vi "Log.vi"(10 "Log Packet":T1, 11 "LVQueue Sink in":refnum<class "LVQueue Sink.lvclass">) -> (0 "error out":errorcluster, 3 "LVQueue Sink out":refnum<class "LVQueue Sink.lvclass">)   [LabVIEW 2019, in "LVQueue Sink.lvclass"]
uses:
  LVQueue Sink.lvclass
  Composed Log/Types/Log Packet.ctl
  Composed Log/Types/Log Level.ctl
  LVQueue Sink.lvclass/LVQueue Sink.ctl
  Composed Log/Composed Log.lvlib
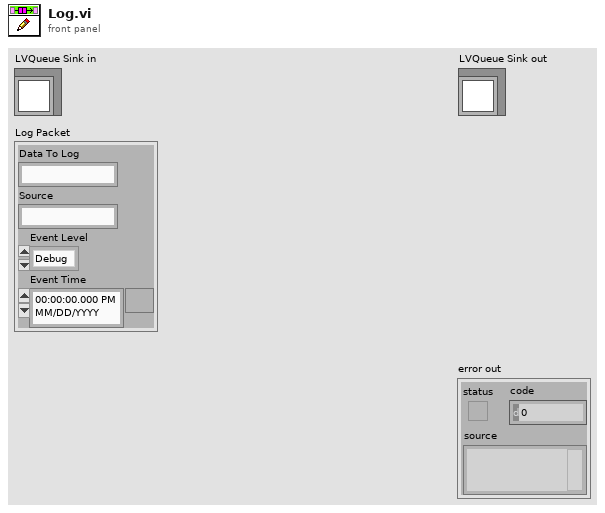
[diagram p1: front panel]
types:
  T1 = typedef "Composed Log.lvlib/Log Packet.ctl" = cluster{"Data To Log":string, "Source":string, "Event Level":T2, "Event Time":timestamp}
  T2 = typedef "Composed Log.lvlib/Log Level.ctl" = enum16{"Debug", "Info", "Warning", "Error", "Critical"}
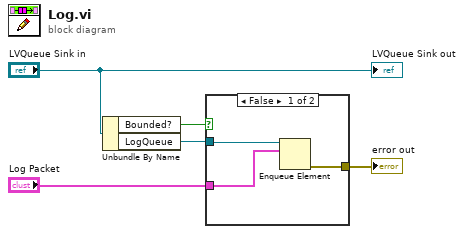
[diagram p0: block diagram]
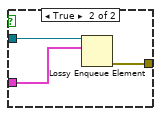
[diagram p2: hidden frame]
diagram:
  n1 = Unbundle By Name("LVQueue Sink in") -> ("Bounded?"=w4:bool, "LogQueue"=w3:refnum<queue>)
  n2 = case shown="False" w4 {
    tunnel: w3 -> [w8 w11]
    tunnel: "Log Packet" -> [w7 w10]
    tunnel: [w6 w9] -> w1
    frame False {
      n3 = Enqueue Element(queue=w8, element=w7) -> (error out=w6:errorcluster)  [unwired: 2 in, 2 out]
    }
    frame True {
      n4 = Lossy Enqueue Element(queue=w11, element=w10) -> (error out=w9:errorcluster)  [unwired: 1 in, 3 out]
    }
  }
  "error out" <- w1
  "LVQueue Sink out" <- "LVQueue Sink in"
